vi "Untitled 3 (SubVI).vi"(10 "X, Y, BEARING in":cluster{dbl, dbl, dbl}, 11 "Queue in":refnum<queue>) -> (2 "X, Y, BEARING out":cluster{dbl, dbl, dbl}, 3 "Queue out":refnum<queue>)   [LabVIEW 2017]
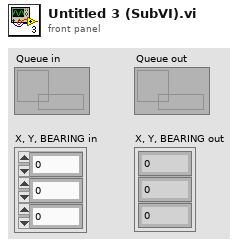
[diagram p1: front panel]
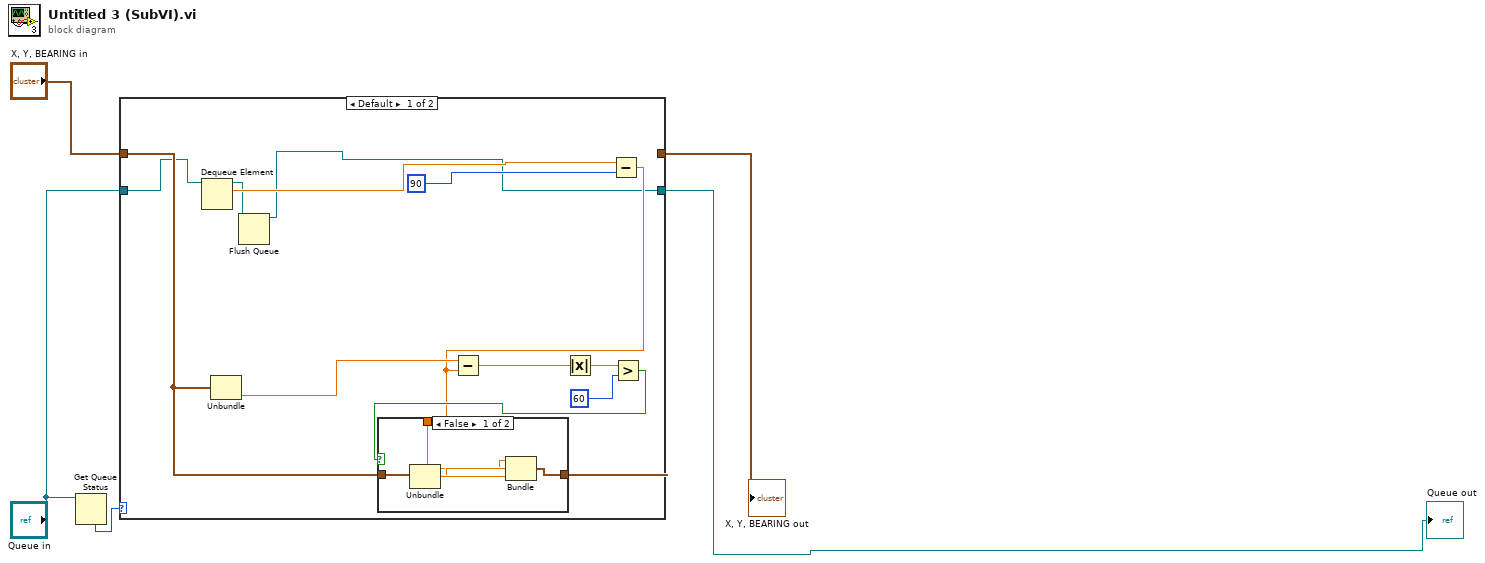
[diagram p0: block diagram]
diagram:
  n1 = Get Queue Status(queue="Queue in") -> (# elements in queue=w1:i32)  [unwired: 2 in, 7 out]
  n2 = case shown="Default" w1 {
    tunnel: "X, Y, BEARING in" -> [w12 w26]
    tunnel: [w13 w26] -> w3
    tunnel: "Queue in" -> [w8 w25]
    tunnel: [w6 w25] -> w5
    frame Default {
      n3 = Dequeue Element(queue=w8) -> (queue out=w7:refnum<queue>, element=w9:dbl)  [unwired: 2 in, 2 out]
      n4 = Unbundle(w12) -> (w11:dbl)  [unwired: 2 out]
      n5 = Flush Queue(queue=w7) -> (queue out=w6:refnum<queue>)  [unwired: 1 in, 2 out]
      n6 = Subtract(x=w9, y=90) -> (x-y=w10:dbl)
      n7 = Subtract(x=w11, y=w10) -> (x-y=w17:dbl)
      n8 = Absolute Value(x=w17) -> (abs(x)=w16:dbl)
      n9 = Greater?(x=w16, y=60) -> (0:w14:bool)
      n10 = case shown="False" w14 {
        tunnel: w12 -> [w23 w24]
        tunnel: [w19 w24] -> w13
        tunnel: w10 -> [w22 _]
        frame False {
          n11 = Unbundle(w23) -> (w20:dbl, w21:dbl)  [unwired: 1 out]
          n12 = Bundle(w20, w21, w22) -> (w19:cluster{dbl, dbl, dbl})  [unwired: 1 in]
        }
        frame True {
        }
      }
    }
    frame 0 {
    }
  }
  "Queue out" <- w5
  "X, Y, BEARING out" <- w3
